vi "EFMC-1.vi"(0 "数组":u8[](array[numeric])) -> (2 "地向速度":i32, 3 "俯仰角":i16, 4 "横滚角":i16, 6 "东向速度":i32, 8 "真航向":i16, 10 "北向速度":i32, 12 "高度":i32, 13 "纬度":i32, 14 "经度":i32)   [LabVIEW 2012]
uses:
  index-i16.vi
  index-i32.vi
  XX-I16.vi
  XX-I32.vi
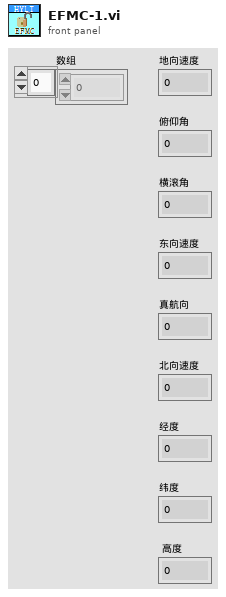
[diagram p1: front panel]
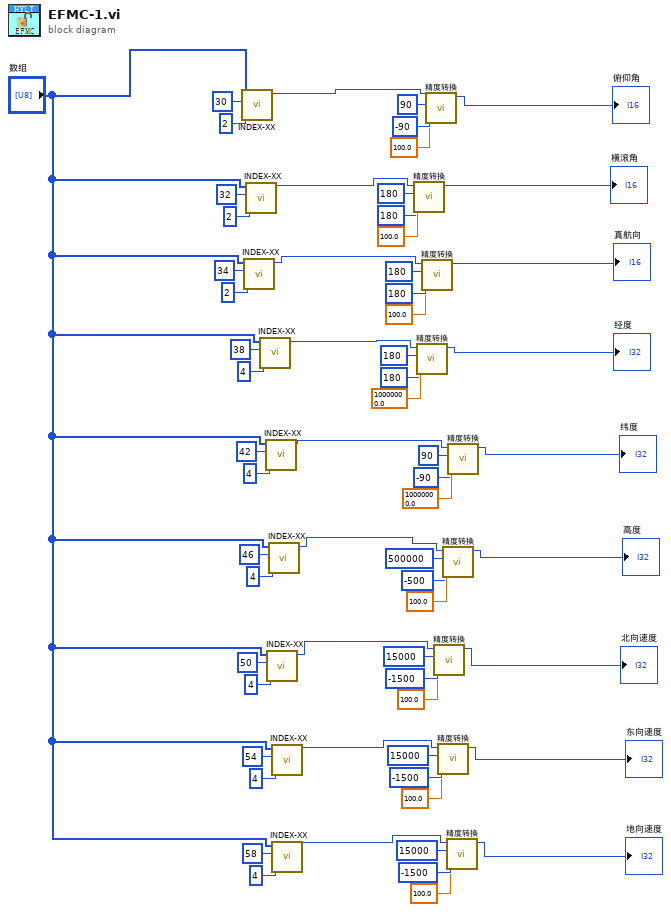
[diagram p0: block diagram]
diagram:
  n1 = call-poly "INDEX-XX.vi"("长度"=2, "索引"=30, "数组"="数组") -> ("数值输出"=w23:i16)  [unwired: 8 in]
  n2 = call-poly "INDEX-XX.vi"("长度"=2, "索引"=34, "数组"="数组") -> ("数值输出"=w33:i16)  [unwired: 8 in]
  n3 = call-poly "INDEX-XX.vi"("长度"=2, "索引"=32, "数组"="数组") -> ("数值输出"=w28:i16)  [unwired: 8 in]
  n4 = call-poly "INDEX-XX.vi"("长度"=4, "索引"=38, "数组"="数组") -> ("数值输出"=w37:i32)  [unwired: 8 in]
  n5 = call-poly "INDEX-XX.vi"("长度"=4, "索引"=42, "数组"="数组") -> ("数值输出"=w46:i32)  [unwired: 8 in]
  n6 = call-poly "INDEX-XX.vi"("长度"=4, "索引"=50, "数组"="数组") -> ("数值输出"=w53:i32)  [unwired: 8 in]
  n7 = call-poly "INDEX-XX.vi"("长度"=4, "索引"=46, "数组"="数组") -> ("数值输出"=w51:i32)  [unwired: 8 in]
  n8 = call-poly "INDEX-XX.vi"("长度"=4, "索引"=54, "数组"="数组") -> ("数值输出"=w58:i32)  [unwired: 8 in]
  n9 = call-poly "INDEX-XX.vi"("长度"=4, "索引"=58, "数组"="数组") -> ("数值输出"=w63:i32)  [unwired: 8 in]
  n10 = call-poly "精度转换.vi"("单位"=100.0, "下限"=i16 180, "上限"=i16 180, "数值输入"=w28) -> ("输出"=→"横滚角":i16)  [unwired: 7 in]
  n11 = call-poly "精度转换.vi"("单位"=10000000.0, "下限"=180, "上限"=180, "数值输入"=w37) -> ("输出"=→"经度":i32)  [unwired: 7 in]
  n12 = call-poly "精度转换.vi"("单位"=100.0, "下限"=i16 180, "上限"=i16 180, "数值输入"=w33) -> ("输出"=→"真航向":i16)  [unwired: 7 in]
  n13 = call-poly "精度转换.vi"("单位"=100.0, "下限"=i16 -90, "上限"=i16 90, "数值输入"=w23) -> ("输出"=→"俯仰角":i16)  [unwired: 7 in]
  n14 = call-poly "精度转换.vi"("单位"=100.0, "下限"=-1500, "上限"=15000, "数值输入"=w53) -> ("输出"=→"北向速度":i32)  [unwired: 7 in]
  n15 = call-poly "精度转换.vi"("单位"=100.0, "下限"=-1500, "上限"=15000, "数值输入"=w58) -> ("输出"=→"东向速度":i32)  [unwired: 7 in]
  n16 = call-poly "精度转换.vi"("单位"=100.0, "下限"=-500, "上限"=500000, "数值输入"=w51) -> ("输出"=→"高度":i32)  [unwired: 7 in]
  n17 = call-poly "精度转换.vi"("单位"=100.0, "下限"=-1500, "上限"=15000, "数值输入"=w63) -> ("输出"=→"地向速度":i32)  [unwired: 7 in]
  n18 = call-poly "精度转换.vi"("单位"=10000000.0, "下限"=-90, "上限"=90, "数值输入"=w46) -> ("输出"=→"纬度":i32)  [unwired: 7 in]
